vi "EOL CAN_Clear_DTC's.vi"(8 "Error in":errorcluster, 10 "Read Session in":refnum<k21>, 11 "Write Session in":refnum<k21>) -> (0 "Error out":errorcluster, 2 "TxRx Data":string[][](array[string]), 3 "Response Good?":bool)   [LabVIEW 2014]
uses:
  <vilib>/xnet/xnet.llb/XNET Frame CAN.ctl
  <vilib>/xnet/xnet.llb/XNET Frame Type CAN.ctl
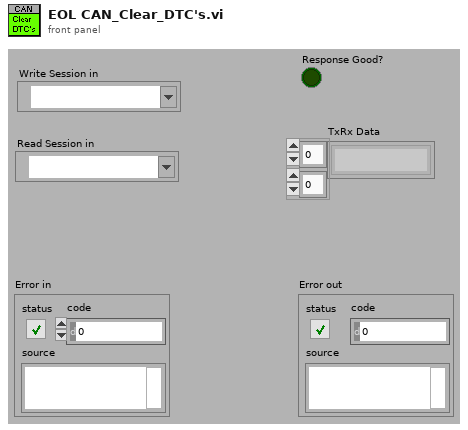
[diagram p1: front panel]
types:
  T1 = typedef "XNET Frame CAN.ctl" = cluster{"timestamp":timestamp, "payload":u8[], "identifier":u32, "type":T2, "extended?":bool, "echo?":bool}
  T2 = typedef "XNET Frame Type CAN.ctl" = u8
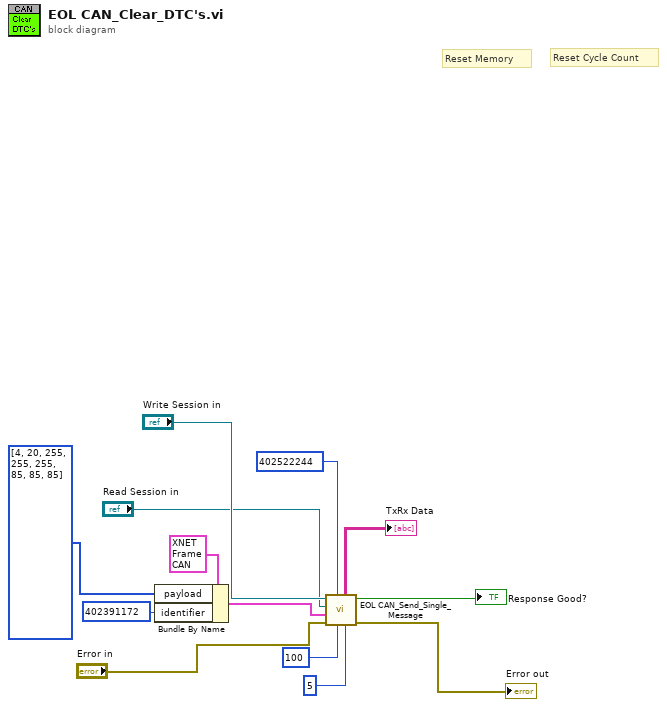
[diagram p0: block diagram]
diagram:
  # "Reset Memory"
  # "Reset Cycle Count"
  n1 = Bundle By Name(cluster=T1 {"timestamp"=timestamp(0 s since 1904-01-01), "payload"=[2, 39, 3, 85, 85, 85, 85, 85], "identifier"=402391172, "type"=8, "extended?"=TRUE, "echo?"=FALSE} ("Tx CAN frame"), "payload"=u8[] [4, 20, 255, 255, 255, 85, 85, 85] ("Transmit Data 2"), "identifier"=u32 402391172) -> (w9:T1)
  n2 = call "EOL CAN_Send_Single_Message.vi"("Retries"=5, "Msg Wait Time"=u32 100, "Rx Arbitration Id"=u32 402522244, "Error in"="Error in", "Tx CAN frame"=w9, "Read Session in"="Read Session in", "Write Session in"="Write Session in") -> ("Error out"=→"Error out":errorcluster, "Response Good?"=→"Response Good?":bool, "TxRx Data"=→"TxRx Data":string[][])  [unwired: 2 out]
